vi "PNG to Pixmap.vi"(11 "path to PNG file":path) -> (1 "Size":string, 3 "String":string)   [LabVIEW 2025]
uses:
  <vilib>/picture/picture.llb/imagedata.ctl
panel:
  out "image data":T1
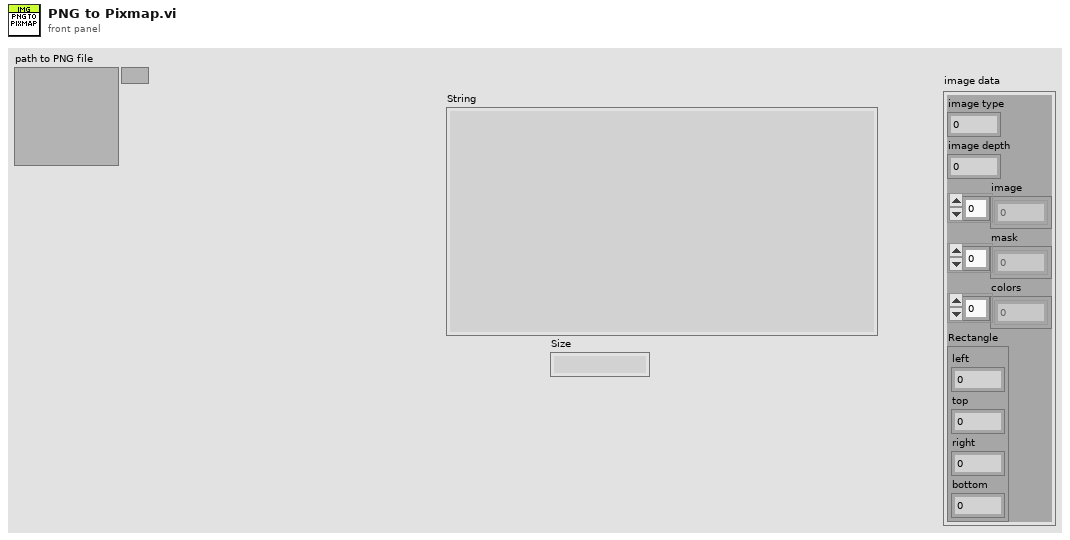
[diagram p1: front panel]
types:
  T1 = typedef "imagedata.ctl" = cluster{"image type":i32, "image depth":i32, "image":u8[], "mask":u8[], "colors":u32[], "Rectangle":cluster{"left":i16, "top":i16, "right":i16, "bottom":i16}}
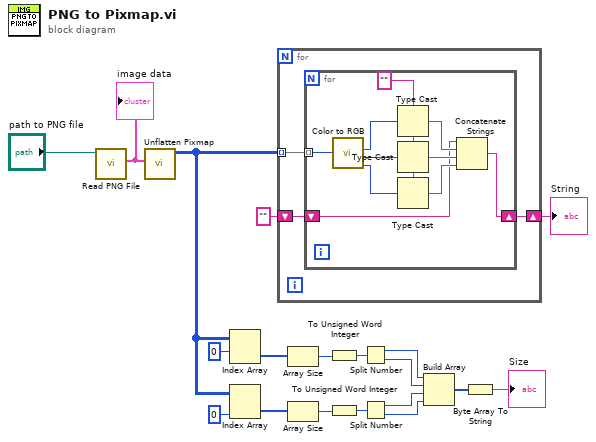
[diagram p0: block diagram]
diagram:
  n1 = call <vilib>:"Read PNG File.vi"("path to PNG file"="path to PNG file") -> ("image data"=w16:T1)  [unwired: 8 in, 2 out]
  "image data" <- w16
  n2 = call <vilib>:"Unflatten Pixmap.vi"("image data"=w16) -> ("24-bit pixmap"=w14:u32[][])  [unwired: 4 in, 6 out]
  n3 = Index Array(array=w14, index (row)=0) -> (element=w12:u32[])  [unwired: 1 in]
  n4 = Index Array(array=w14, index (col)=0 ("disabled index (col)")) -> (element=w11:u32[])  [unwired: 1 in]
  n5 = for {
    tunnel: w14 -> [w22] mode=indexing
    shift-right: [w21] -> w17
    shift-left: "" -> [w20]
    n6 = for {
      tunnel: w22 -> [w32] mode=indexing
      shift-right: [w24] -> w21
      shift-left: w20 -> [w23]
      w28 = "" ("type")
      n7 = call <vilib>:"Color to RGB.vi"("Color"=w32) -> ("R"=w31:u8, "G"=w30:u8, "B"=w29:u8)  [unwired: 1 out]
      n8 = Type Cast(type=w28, x=w31) -> (*(type *) &x=w26:string)
      n9 = Type Cast(type=w28, x=w30) -> (*(type *) &x=w27:string)
      n10 = Type Cast(type=w28, x=w29) -> (*(type *) &x=w25:string)
      n11 = Concatenate Strings(w23, w26, w27, w25) -> (w24:string)
    }
  }
  "String" <- w17
  n12 = Array Size(array=w12) -> (size(s)=w9:i32)
  n13 = Array Size(array=w11) -> (size(s)=w10:i32)
  n14 = To Unsigned Word Integer(number=w9) -> (unsigned 16bit integer=w8:u16)
  n15 = To Unsigned Word Integer(number=w10) -> (unsigned 16bit integer=w7:u16)
  n16 = Split Number(x=w8) -> (hi(x)=w4:u8, lo(x)=w3:u8)
  n17 = Split Number(x=w7) -> (hi(x)=w5:u8, lo(x)=w6:u8)
  n18 = Build Array(w4, w3, w5, w6) -> (w2:u8[])
  n19 = Byte Array To String(unsigned byte array=w2) -> (string=→"Size":string)
